vi "NISE.local.Read Dev.CapsVersion.vi"(8 "error in (no error)":errorcluster, 11 "SLSC Local in":refnum<class "SLSC Interface.lvclass">) -> (0 "error out":errorcluster, 2 "Dev.CapsVersion":string, 3 "SLSC Local out":refnum<class "SLSC Interface.lvclass">)   [LabVIEW 2016, in "SLSC Interface.lvclass"]
uses:
  SLSC Interface Class/SLSC Interface.lvclass
  SLSC Interface Class/NISE.Read session.vi
  <resource>/objmgr/slsc.rc
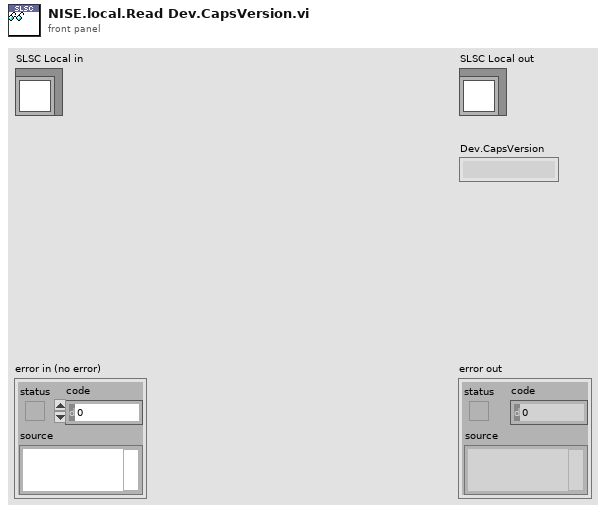
[diagram p1: front panel]
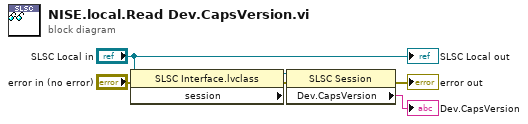
[diagram p0: block diagram]
diagram:
  n1 = property class="SLSC Interface.lvclass"(reference="SLSC Local in", error in="error in (no error)") -> (error out=w2:errorcluster, "session"=w5:refnum<k21>)  [unwired: 1 out]
  n2 = property class="SLSC Session"(reference=w5, error in=w2) -> (error out=→"error out":errorcluster, "Dev.CapsVersion"=→"Dev.CapsVersion":string)  [unwired: 1 out]
  "SLSC Local out" <- "SLSC Local in"
